vi "Layout - Parse VI for String Control Reference.vi"(8 "error in (no error)":errorcluster, 10 "String Label":string, 11 "VI in":refnum<vi>) -> (0 "error out":errorcluster, 3 "String Reference":refnum<vi>)   [LabVIEW 2020, in "UI Manager.lvlib"]
doc: "Parses the <b>VI in</b> for a string control labelled <b>String Label</b> and returns the reference to it.\n\n____\nHAMPEL SOFTWARE ENGINEERING v2.6.0 (2023-12-19 10:54)"
uses:
  UI Manager.lvlib
  <vilib>/Utility/traverseref.llb/TRef TravTarget.ctl
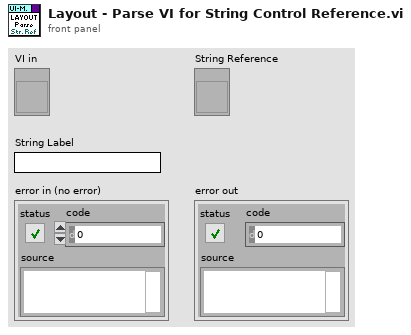
[diagram p1: front panel]
types:
  T1 = typedef "TRef TravTarget.ctl" = enum16{"FP", "BD", "Other"}
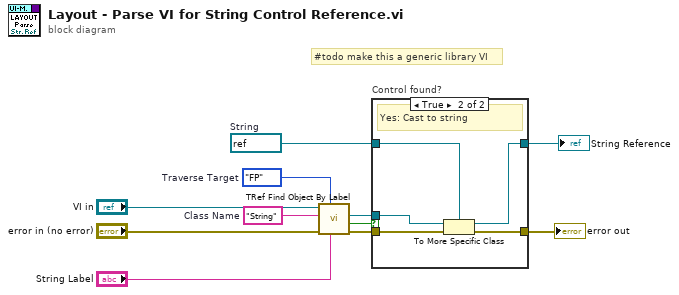
[diagram p0: block diagram]
diagram:
  w7 = refnum<vi> refnum  # String
  w4 = TRef_TravTarget."FP"  # Traverse Target
  w3 = "String"  # Class Name
  # "#todo make this a generic library VI"
  n1 = call <vilib>:"TRef Find Object By Label.vi"("Label"="String Label", "Traverse Target"=w4, "error in (no error)"="error in (no error)", "Class Name"=w3, "VI Ref"="VI in") -> ("error out"=w6:errorcluster, "Found?"=w1:bool, "Found Obj Ref"=w5:refnum<vi>)  [unwired: 3 in, 1 out]
  n2 = case "Control found?" shown="True" w1 {
    tunnel: [w12 w18] -> w11
    tunnel: w7 -> [w13 w17]
    tunnel: w6 -> [w12 w16]
    tunnel: w5 -> [_ w15]
    tunnel: [w13 w14] -> w2
    frame False {
      # "No: Do nothing"
    }
    frame True {
      # "Yes: Cast to string"
      n3 = To More Specific Class(target class=w17, reference=w15, error in=w16) -> (specific class reference=w14:refnum<vi>, error out=w18:errorcluster)
    }
  }
  "error out" <- w11
  "String Reference" <- w2
